vi "Outgoing Page.vi"(8 "error in (no error)":errorcluster, 11 "Node Ptr":T2 format="%.0x") -> (0 "error out":errorcluster)   [LabVIEW 2023, in "Protection and Counter Addon System Explorer.lvlib"]
uses:
  Protection and Counter Addon System Explorer.lvlib
  <vilib>/NI VeriStand/Custom Device API/Custom Device Item Ref.ctl
  SubModules/Frame-Protection-Support/Source/Shared/Types/Protection Type.ctl
  SubModules/Frame-Protection-Support/Source/System Explorer/Types/Auto Config Setting.ctl
  Addon Shared/SubVIs/GUID Lookup.vi
  <vilib>/NI VeriStand/Custom Device API/Get Item Property (Variant).vi
  <vilib>/NI VeriStand/Custom Device API/Set Item Property (Variant).vi
  <vilib>/NI VeriStand/Custom Device API/Custom Device API.lvlib
  Addon Shared/Protection and Counter Addon Shared.lvlib
  SubModules/Frame-Protection-Support/Source/System Explorer/Protection and Counter Support System Explorer.lvlib
  SubModules/Frame-Protection-Support/Source/Shared/Protection and Counter Support Shared.lvlib
panel:
  in  "Rolling Counter Max Count":dbl=15.0
  in  "Protection Type":T1=enum."LP_CRC8"
  in  "Commit":bool
  in  "CRC Matching Strings":string[](array[string])
  in  "RC Matching Strings":string[](array[string])
  in  "CRC":bool
  in  "Rolling Counter":bool
  in  "SHDocVw.IWebBrowser":refnum<k7>(container)
  in  "Header":cluster{"Section Name":string}={"Section Name"="Auto Config Settings"}
  out "Name":string
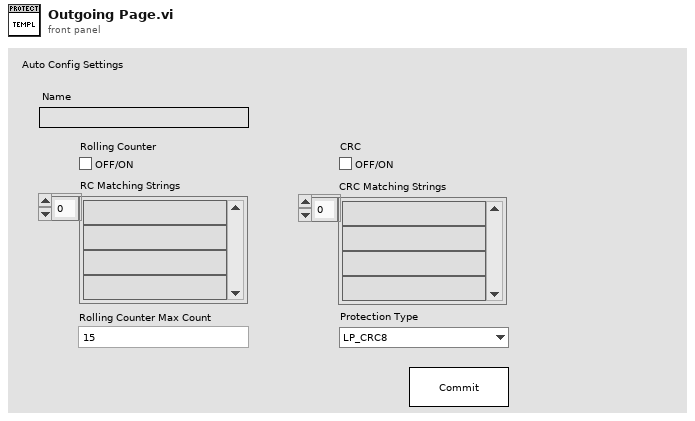
[diagram p1: front panel]
types:
  T1 = typedef "Protection and Counter Support Shared.lvlib/Protection Type.ctl" = enum16{"Arb ID + Bytes Checksum with Inversion", "Arb ID + Bytes CRC with Inversion", "Reversed Raw Signal Checksum with Inversion", "Concatenated Two's Compliment", "LP_CRC8", "LP_Checksum", "LP_CRC8_MRS"}
  T2 = typedef "Custom Device API.lvlib/Custom Device Item Ref.ctl" = u64
  T3 = typedef "Protection and Counter Support System Explorer.lvlib/Auto Config Setting.ctl" = cluster{"Rolling Counter":bool, "RC Matching Strings":string[], "CRC":bool, "CRC Matching Strings":string[], "Rolling Counter Max Count":dbl, "Protection Type Number":u8}
  T4 = typedef "Custom Device API.lvlib/Custom Device Item Info.ctl" = cluster{"Name":string, "Is Channel":bool, "GUID":string, "Is Waveform":bool}
  T5 = typedef "Custom Device API.lvlib/Custom Device Commands.ctl" = enum16{"Default", "Item renamed", "Shutdown", "Dynamic button pressed"}
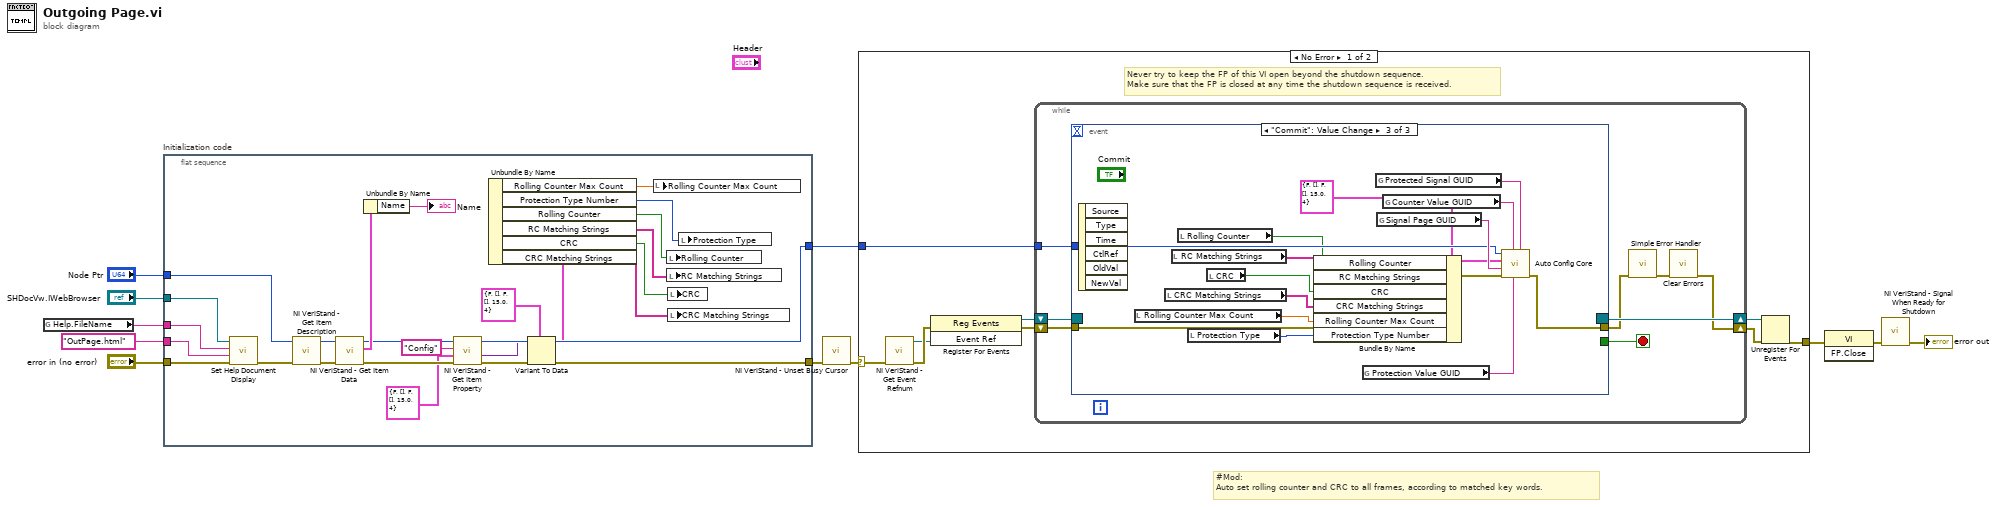
[diagram p0: block diagram]
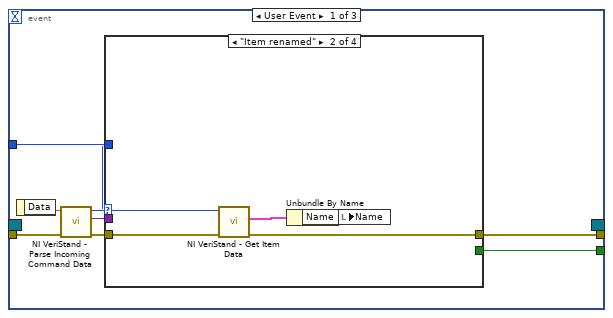
[diagram p2: hidden frame]
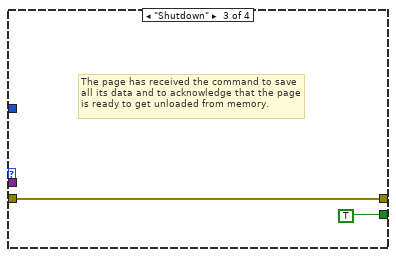
[diagram p4: hidden frame]
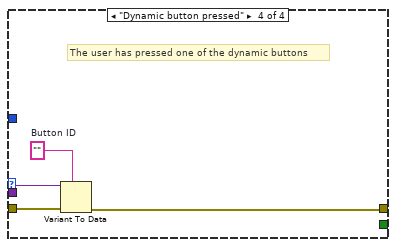
[diagram p5: hidden frame]
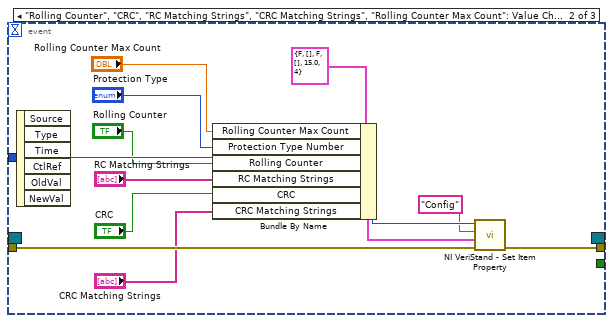
[diagram p6: hidden frame]
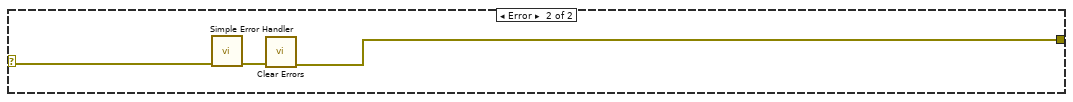
[diagram p7: hidden frame]
diagram:
  # "#Mod:\nAuto set rolling counter and CRC to all frames, according to matched key words."
  n1 = global read "GUID Lookup.vi" "Help.FileName"() -> (w1:string)
  n2 = flat-sequence "Initialization code" {
    tunnel: "error in (no error)" -> [w32]
    tunnel: "Node Ptr" -> [w36]
    tunnel: [w22] -> w7
    tunnel: [w25] -> w4
    tunnel: "OutPage.html" ("HTML File") -> [w30]
    tunnel: w1 -> [w29]
    tunnel: "SHDocVw.IWebBrowser" -> [w28]
    frame #0 {
      n3 = call "Set Help Document Display.vi"("error in (no error)"=w32, "HTML File"=w30, "Main CHM File"=w29, "SHDocVw.IWebBrowser2"=w28) -> ("error out"=w31:errorcluster)  [unwired: 7 in]
      n4 = call <vilib>:"NI VeriStand - Get Item Description.vi"("error in (no error)"=w31, "Item Ref in"=w36) -> ("error out"=w35:errorcluster, "Item Ref out"=w37:T2)  [unwired: 8 out]
      n5 = call <vilib>:"NI VeriStand - Get Item Data.vi"("error in (no error)"=w35, "Item Ref in"=w37) -> ("error out"=w26:errorcluster, "Item Info"=w34:T4, "Item Ref out"=w27:T2)  [unwired: 7 out]
      n6 = Unbundle By Name(w34) -> ("Name"=→"Name":string)
      n7 = call-poly <vilib>:"NI VeriStand - Get Item Property.vi"("error in (no error)"=w26, "Default Value"=T3 {"Rolling Counter"=FALSE, "RC Matching Strings"=[], "CRC"=FALSE, "CRC Matching Strings"=[], "Rolling Counter Max Count"=15.0, "Protection Type Number"=4} ("Auto Config Setting"), "Property Name"="Config", "Item Ref in"=w27) -> ("error out"=w23:errorcluster, "Value"=w20:variant, "Item Ref out"=w25:T2)  [unwired: 4 in, 1 out]
      n8 = Variant To Data(error in=w23, type=T3 {"Rolling Counter"=FALSE, "RC Matching Strings"=[], "CRC"=FALSE, "CRC Matching Strings"=[], "Rolling Counter Max Count"=15.0, "Protection Type Number"=4} ("Auto Config Setting"), Variant=w20) -> (data=w19:T3, error out=w22:errorcluster)
      n9 = Unbundle By Name(w19) -> ("Rolling Counter Max Count"=w13:dbl, "Protection Type Number"=w12:u8, "Rolling Counter"=w18:bool, "RC Matching Strings"=w17:string[], "CRC"=w16:bool, "CRC Matching Strings"=w15:string[])
      n10 = local write "Rolling Counter Max Count"(w13) -> ()
      n11 = local write "Rolling Counter"(w18) -> ()
      n12 = local write "RC Matching Strings"(w17) -> ()
      n13 = local write "CRC"(w16) -> ()
      n14 = local write "CRC Matching Strings"(w15) -> ()
      n15 = local write "Protection Type"(w12) -> ()
    }
  }
  n16 = call <vilib>:"NI VeriStand - Unset Busy Cursor.vi"("error in (no error)"=w7) -> ("error out"=w6:errorcluster)  [unwired: 10 out]
  n17 = case shown="No Error" w6 {
    selector: w6 -> [w38 w104]
    tunnel: [w43 w102] -> w11
    tunnel: w4 -> [w39 _]
    frame No Error {
      # "Never try to keep the FP of this VI open beyond the shutdown sequence.\nMake sure that the FP is closed at any time the shutdown sequence is received."
      n18 = call <vilib>:"NI VeriStand - Get Event Refnum.vi"("error in (no error)"=w38) -> ("error out"=w46:errorcluster, "Event Ref"=w42:refnum<user-event>)  [unwired: 9 out]
      n19 = register-events(error in=w46, w42) -> (reference out=w40:refnum<event-registration>, error out=w41:errorcluster)  [unwired: 1 in]
      n20 = while {
        tunnel: w39 -> [w50]
        shift-right: [w47] -> w44
        shift-left: w41 -> [w53]
        shift-right: [w54] -> w45
        shift-left: w40 -> [w52]
        stop <- w51 stop-if-true
        n21 = event shown="[2] \"Commit\": Value Change" {
          selector: w52 -> [_ _ _]
          dyn-events: [_ _ _] -> w54
          timeout: _ -> [_ _ _]
          tunnel: w53 -> [w62 w85 w97]
          tunnel: [w58 _ _] -> w51
          tunnel: [w57 w84 w98] -> w49
          tunnel: w50 -> [w56 w86 w96]
          event User Event {
            n22 = event-data() -> ("Data"=w61:string)  [unwired: 1 out]
            n23 = call <vilib>:"NI VeriStand - Parse Incoming Command Data.vi"("error in (no error)"=w62, "Incoming data"=w61) -> ("error out"=w60:errorcluster, "Outgoing data"=w55:variant, "Action"=w59:T5)  [unwired: 7 out]
            n24 = case shown="\"Item renamed\"" w59 {
              tunnel: w60 -> [w63 w68 w69 w74]
              tunnel: [_ _ TRUE _] -> w58
              tunnel: [w63 w65 w69 w71] -> w57
              tunnel: w56 -> [_ w67 _ _]
              tunnel: w55 -> [_ _ _ w73]
              frame "Default", Default {
              }
              frame "Item renamed" {
                n25 = call <vilib>:"NI VeriStand - Get Item Data.vi"("error in (no error)"=w68, "Item Ref in"=w67) -> ("error out"=w65:errorcluster, "Item Info"=w66:T4)  [unwired: 8 out]
                n26 = Unbundle By Name(w66) -> ("Name"=w64:string)
                n27 = local write "Name"(w64) -> ()
              }
              frame "Shutdown" {
                # "The page has received the command to save all its data and to acknowledge that the page is ready to get unloaded from memory."
              }
              frame "Dynamic button pressed" {
                w72 = ""  # Button ID
                # "The user has pressed one of the dynamic buttons"
                n28 = Variant To Data(error in=w74, type=w72, Variant=w73) -> (error out=w71:errorcluster)  [unwired: 1 out]
              }
            }
          }
          event "Rolling Counter", "CRC", "RC Matching Strings", "CRC Matching Strings", "Rolling Counter Max Count": Value Change {
            n29 = event-data() -> ()  [unwired: 7 out]
            n30 = Bundle By Name(cluster=T3 {"Rolling Counter"=FALSE, "RC Matching Strings"=[], "CRC"=FALSE, "CRC Matching Strings"=[], "Rolling Counter Max Count"=15.0, "Protection Type Number"=4} ("Auto Config Setting"), "Rolling Counter Max Count"="Rolling Counter Max Count", "Protection Type Number"="Protection Type", "Rolling Counter"="Rolling Counter", "RC Matching Strings"="RC Matching Strings", "CRC"="CRC", "CRC Matching Strings"="CRC Matching Strings") -> (w77:T3)
            n31 = call-poly <vilib>:"NI VeriStand - Set Item Property.vi"("error in (no error)"=w85, "Value"=w77, "Property Name"="Config", "Item Ref in"=w86) -> ("error out"=w84:errorcluster)  [unwired: 5 in, 2 out]
          }
          event "Commit": Value Change {
            n32 = event-data() -> ()  [unwired: 7 out]
            n33 = local read "Rolling Counter Max Count"() -> (w88:dbl)
            n34 = local read "CRC Matching Strings"() -> (w91:string[])
            n35 = local read "RC Matching Strings"() -> (w93:string[])
            n36 = local read "Rolling Counter"() -> (w95:bool)
            n37 = local read "Protection Type"() -> (w87:T1)
            n38 = local read "CRC"() -> (w92:bool)
            n39 = Bundle By Name(cluster=T3 {"Rolling Counter"=FALSE, "RC Matching Strings"=[], "CRC"=FALSE, "CRC Matching Strings"=[], "Rolling Counter Max Count"=15.0, "Protection Type Number"=4} ("Auto Config Setting"), "Rolling Counter"=w95, "RC Matching Strings"=w93, "CRC"=w92, "CRC Matching Strings"=w91, "Rolling Counter Max Count"=w88, "Protection Type Number"=w87) -> (w90:T3)
            n40 = global read "GUID Lookup.vi" "Protection Value GUID"() -> (w89:string)
            n41 = global read "GUID Lookup.vi" "Protected Signal GUID"() -> (w99:string)
            n42 = global read "GUID Lookup.vi" "Signal Page GUID"() -> (w101:string)
            n43 = global read "GUID Lookup.vi" "Counter Value GUID"() -> (w100:string)
            n44 = call "Auto Config Core.vi"("Protected Signal GUID"=w99, "Protection Value GUID"=w89, "Counter Value GUID"=w100, "error in (no error)"=w97, "Signal Page GUID"=w101, "Auto Config Setting"=w90, "Node Ptr"=w96) -> ("error out"=w98:errorcluster)  [unwired: 4 in]
          }
        }
        n45 = call <vilib>:"Simple Error Handler.vi"("error in (no error)"=w49) -> ("error out"=w48:errorcluster)  [unwired: 1 in, 7 out]
        n46 = call <vilib>:"Clear Errors.vi"("error in (no error)"=w48) -> ("error out"=w47:errorcluster)  [unwired: 1 in, 5 out]
      }
      n47 = Unregister For Events(event registration refnum=w45, error in=w44) -> (error out=w43:errorcluster)
    }
    frame Error {
      n48 = call <vilib>:"Simple Error Handler.vi"("error in (no error)"=w104) -> ("error out"=w103:errorcluster)  [unwired: 1 in, 7 out]
      n49 = call <vilib>:"Clear Errors.vi"("error in (no error)"=w103) -> ("error out"=w102:errorcluster)  [unwired: 1 in, 5 out]
    }
  }
  n50 = invoke class="VI" method="FP.Close"(error in=w11) -> (error out=w10:errorcluster)  [unwired: 2 in, 2 out]
  n51 = call <vilib>:"NI VeriStand - Signal When Ready for Shutdown.vi"("error in (no error)"=w10) -> ("error out"=→"error out":errorcluster)  [unwired: 10 out]
